vi "Set Server gRPC UEs.vi"(10 "Server gRPC UEs":T1, 11 "OOP Server in":refnum<class "HVC8.lvclass">) -> (3 "OOP Server out":refnum<class "HVC8.lvclass">)   [LabVIEW 2019, in "HVC8.lvlib" / "HVC8.lvclass"]
uses:
  HVC8.lvclass
  typeDefs/Server gRPC UEs.ctl
  gRPC lvSupport/Server API/typeDefs/gRPCId Cluster.ctl
  gRPC lvSupport/Server API/typeDefs/grpcId.ctl
  HVC8.lvclass/HVC8.ctl
  gRPC lvSupport/gprc-lvsupport.lvlib
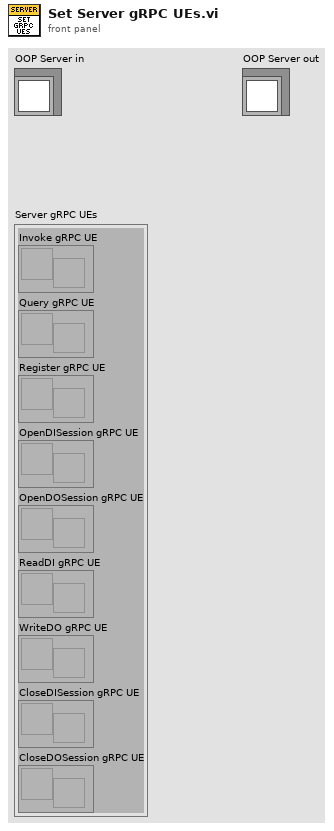
[diagram p1: front panel]
types:
  T1 = typedef "HVC8.lvlib/HVC8.lvclass/Server gRPC UEs.ctl" = cluster{"Invoke gRPC UE":refnum<user-event>, "Query gRPC UE":refnum<user-event>, "Register gRPC UE":refnum<user-event>, "OpenDISession gRPC UE":refnum<user-event>, "OpenDOSession gRPC UE":refnum<user-event>, "ReadDI gRPC UE":refnum<user-event>, "WriteDO gRPC UE":refnum<user-event>, "CloseDISession gRPC UE":refnum<user-event>, "CloseDOSession gRPC UE":refnum<user-event>}
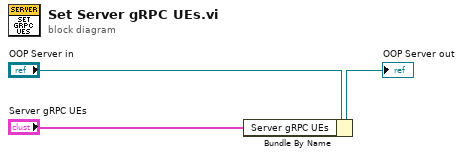
[diagram p0: block diagram]
diagram:
  n1 = Bundle By Name(cluster="OOP Server in", "Server gRPC UEs"="Server gRPC UEs") -> (→"OOP Server out":refnum<class "HVC8.lvclass">)
